vi "Convert Volts to Num.vi"(1 "Numeric":dbl) -> (0 "String":string)   [LabVIEW 2013]
panel:
  out "Numeric (SI Notation)":dbl format="%#_6p"
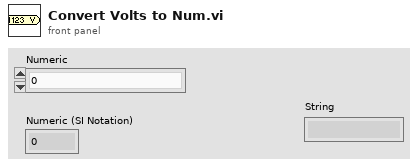
[diagram p1: front panel]
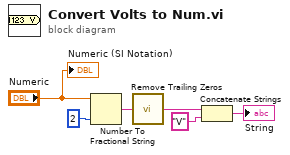
[diagram p0: block diagram]
diagram:
  n1 = Number To Fractional String(number="Numeric", precision (6)=i16 2) -> (F-format string=w5:string)  [unwired: 2 in]
  n2 = call "Remove Trailing Zeros.vi"("String In"=w5) -> ("String Out"=w6:string)
  n3 = Concatenate Strings(w6, "V" ("string")) -> (→"String":string)
  "Numeric (SI Notation)" <- "Numeric"
